vi "KE622x -- 2182 -A Get Digital Filter Count.vi"(0 "622x Resource In":refnum<visa-resource-name>, 1 "Check For SCPI Errors? (T)":bool=TRUE, 11 "error in (no error)":errorcluster) -> (4 "622x Resource Out (dupl)":refnum<visa-resource-name>, 8 "Filter Count":u32=1, 15 "error out":errorcluster)   [LabVIEW 2013, in "Keithly user program.lvlib"]
uses:
  Keithly user program.lvlib
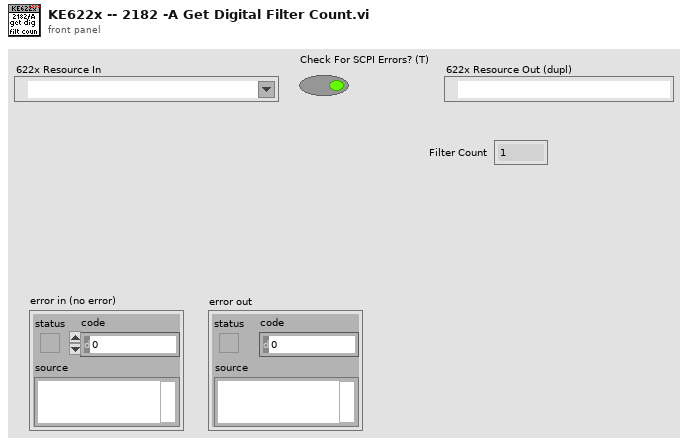
[diagram p1: front panel]
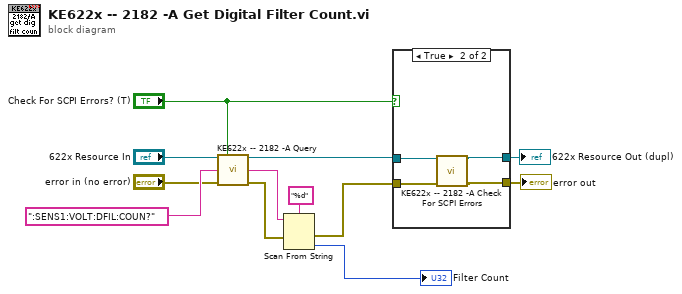
[diagram p0: block diagram]
diagram:
  n1 = call "KE622x -- 2182 -A Query.vi"("622x Resource In"="622x Resource In", "Check For SCPI Errors? (T)"="Check For SCPI Errors? (T)", "2182-A Write String"=":SENS1:VOLT:DFIL:COUN?", "error in (no error)"="error in (no error)") -> ("622x Resource Out (dupl)"=w6:refnum<visa-resource-name>, "2182-A Reponse String"=w4:string, "error out"=w1:errorcluster)  [unwired: 9 in]
  n2 = Scan From String(format string="%d", input string=w4, error in=w1) -> (error out=w11:errorcluster, output 1=→"Filter Count":u32)  [unwired: 2 in, 2 out]
  n3 = case shown="True" "Check For SCPI Errors? (T)" {
    tunnel: w6 -> [w14 w18]
    tunnel: w11 -> [w13 w16]
    tunnel: [w14 w17] -> w10
    tunnel: [w13 w15] -> w9
    frame False {
    }
    frame True {
      n4 = call "KE622x -- 2182 -A Check For SCPI Errors.vi"("VISA Resource In"=w18, "error in (no error)"=w16) -> ("VISA Resource Out (dupl)"=w17:refnum<visa-resource-name>, "error out"=w15:errorcluster)  [unwired: 10 in, 2 out]
    }
  }
  "622x Resource Out (dupl)" <- w10
  "error out" <- w9
